vi "Focus RGB Image Stack.vi"(4 "Height Map":T1, 6 "Focused Image":T1, 8 "error in (no error)":errorcluster, 10 "Kernel Size":i32, 11 "Image Stack":T1[](array[typedef])) -> (0 "error out":errorcluster, 2 "Height Map":T1(plugin-control), 3 "Focused Image":T1(plugin-control))   [LabVIEW 2013]
uses:
  <vilib>/vision/Image Controls.llb/IMAQ Image.ctl
  <vilib>/vision/NI_Vision_Development_Module.lvlib
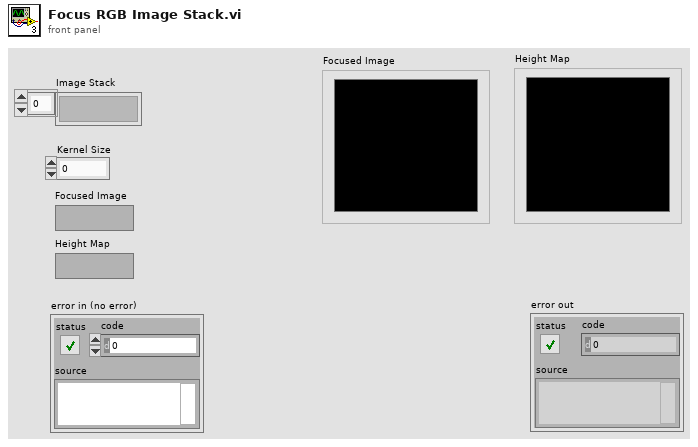
[diagram p1: front panel]
types:
  T1 = typedef "IMAQ Image.ctl" = refnum<image>
  T2 = typedef "Image Type" = u32
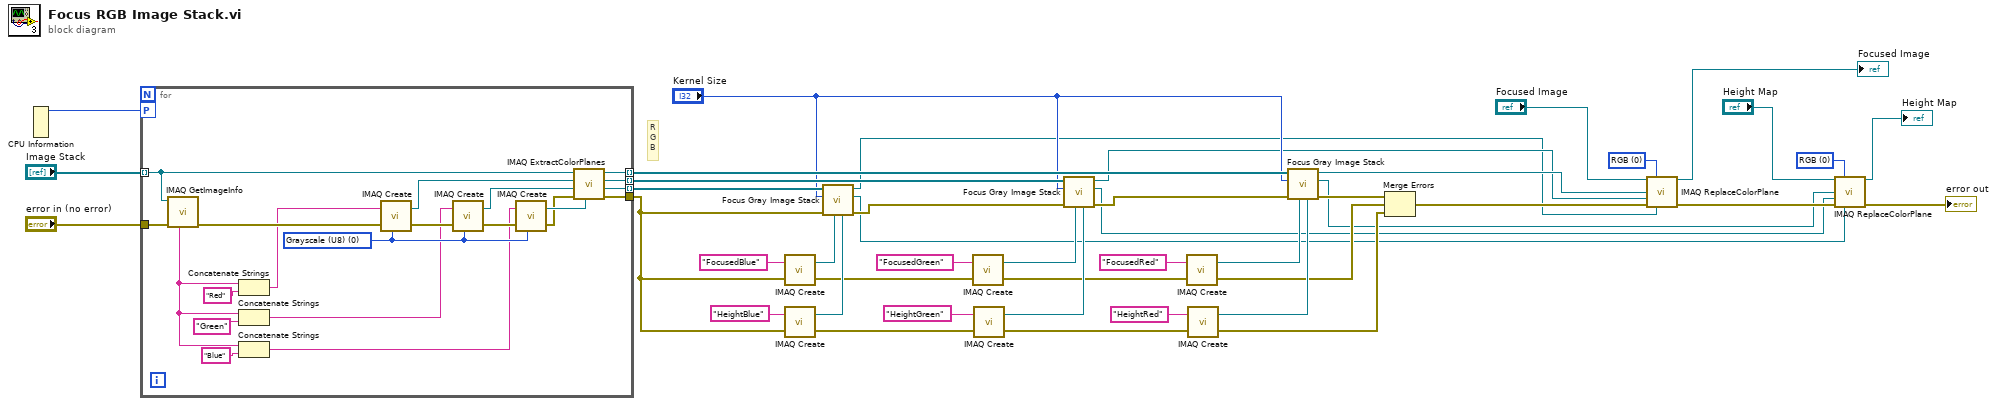
[diagram p0: block diagram]
diagram:
  w37 = u16 0 items=["RGB", "HSL", "HSV", "HSI"] ("Color Mode")
  w41 = u16 0 items=["RGB", "HSL", "HSV", "HSI"] ("Color Mode")
  # "R\nG\nB"
  n1 = CPU Information() -> (4:w42:i32)  [unwired: 3 out]
  n2 = for {
    tunnel: "Image Stack" -> [w45] mode=indexing
    tunnel: "error in (no error)" -> [w65]
    tunnel: [w49] -> w36 mode=indexing
    tunnel: [w48] -> w38 mode=indexing
    tunnel: [w47] -> w40 mode=indexing
    tunnel: [w46] -> w30
    workers-P: w42 -> [_]
    w56 = T2 0 items=["Grayscale (U8)", "Grayscale (I16)", "Grayscale (SGL)", "Complex (CSG)", "RGB (U32)", "HSL (U32)", "RGB (U64)", "Grayscale (U16)"] ("Image Type")
    n3 = call "IMAQ GetImageInfo"("error in (no error)"=w65, "Image"=w45) -> ("error out"=w60:errorcluster, "Image Name"=w64:string)  [unwired: 2 in, 6 out]
    n4 = Concatenate Strings(w64, "Red" ("string")) -> (w57:string)
    n5 = Concatenate Strings(w64, "Green" ("string")) -> (w54:string)
    n6 = Concatenate Strings(w64, "Blue" ("string")) -> (w55:string)
    n7 = call "IMAQ Create"("Image Name"=w57, "Image Type"=w56, "error in (no error)"=w60) -> ("New Image"=w53:T1, "error out"=w59:errorcluster)  [unwired: 2 in]
    n8 = call "IMAQ Create"("Image Name"=w54, "Image Type"=w56, "error in (no error)"=w59) -> ("New Image"=w52:T1, "error out"=w58:errorcluster)  [unwired: 2 in]
    n9 = call "IMAQ Create"("Image Name"=w55, "Image Type"=w56, "error in (no error)"=w58) -> ("New Image"=w51:T1, "error out"=w50:errorcluster)  [unwired: 2 in]
    n10 = call "IMAQ ExtractColorPlanes"("Blue or Luma or Val or Inten Plane"=w51, "error in (no error)"=w50, "Green or Sat Plane"=w52, "Red or Hue Plane"=w53, "Image Src"=w45) -> ("error out"=w46:errorcluster, "Blue or Luma or Val or Inten Plane out"=w47:T1, "Green or Sat Plane out"=w48:T1, "Red or Hue Plane out"=w49:T1)  [unwired: 3 in]
  }
  n11 = call "IMAQ Create"("Image Name"="FocusedBlue", "error in (no error)"=w30) -> ("New Image"=w34:T1, "error out"=w28:errorcluster)  [unwired: 3 in]
  n12 = call "IMAQ Create"("Image Name"="HeightBlue", "error in (no error)"=w30) -> ("New Image"=w31:T1, "error out"=w26:errorcluster)  [unwired: 3 in]
  n13 = call "Focus Gray Image Stack.vi"("Height Map"=w31, "Focused Image"=w34, "error in (no error)"=w30, "Kernel Size"="Kernel Size", "Image Stack"=w40) -> ("error out"=w39:errorcluster, "Height Map"=w6:T1, "Focused Image"=w9:T1)  [unwired: 4 in]
  n14 = call "IMAQ Create"("Image Name"="FocusedGreen", "error in (no error)"=w28) -> ("New Image"=w25:T1, "error out"=w23:errorcluster)  [unwired: 3 in]
  n15 = call "IMAQ Create"("Image Name"="HeightGreen", "error in (no error)"=w26) -> ("New Image"=w24:T1, "error out"=w22:errorcluster)  [unwired: 3 in]
  n16 = call "Focus Gray Image Stack.vi"("Height Map"=w24, "Focused Image"=w25, "error in (no error)"=w39, "Kernel Size"="Kernel Size", "Image Stack"=w38) -> ("error out"=w35:errorcluster, "Height Map"=w7:T1, "Focused Image"=w10:T1)  [unwired: 4 in]
  n17 = call "IMAQ Create"("Image Name"="FocusedRed", "error in (no error)"=w23) -> ("New Image"=w19:T1, "error out"=w16:errorcluster)  [unwired: 3 in]
  n18 = call "IMAQ Create"("Image Name"="HeightRed", "error in (no error)"=w22) -> ("New Image"=w18:T1, "error out"=w15:errorcluster)  [unwired: 3 in]
  n19 = call "Focus Gray Image Stack.vi"("Height Map"=w18, "Focused Image"=w19, "error in (no error)"=w35, "Kernel Size"="Kernel Size", "Image Stack"=w36) -> ("error out"=w17:errorcluster, "Height Map"=w8:T1, "Focused Image"=w11:T1)  [unwired: 4 in]
  n20 = Merge Errors(w17, w16, w15) -> (w13:errorcluster)
  n21 = call "IMAQ ReplaceColorPlane"("Image Src"="Focused Image", "Color Mode"=w37, "Red or Hue Plane"=w11, "Green or Sat Plane"=w10, "error in (no error)"=w13, "Blue or Luma or Val or Inten Plane"=w9) -> ("Image Dst Out"=→"Focused Image":T1, "error out"=w12:errorcluster)  [unwired: 8 in]
  n22 = call "IMAQ ReplaceColorPlane"("Image Src"="Height Map", "Color Mode"=w41, "Red or Hue Plane"=w8, "Green or Sat Plane"=w7, "error in (no error)"=w12, "Blue or Luma or Val or Inten Plane"=w6) -> ("Image Dst Out"=→"Height Map":T1, "error out"=→"error out":errorcluster)  [unwired: 8 in]
